vi "Example Indicator.vi"() -> ()   [LabVIEW 2010]
uses:
  C:/tf/play/labview/Tinkerforge.dll
  Tinkerforge.dll
panel:
  in  "uid":string="amb"
  in  "port":i32=4223
  in  "host":string="localhost"
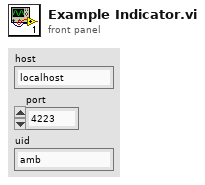
[diagram p1: front panel]
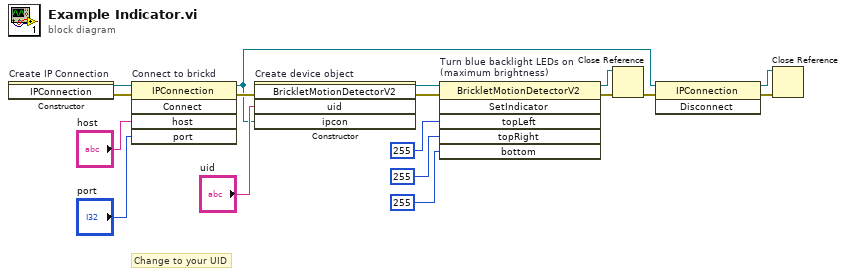
[diagram p0: block diagram]
diagram:
  # "Change to your UID"
  n1 = constructor on="Create IP Connection" class="IPConnection"() -> (reference out=w17:refnum<k24>, error out=w4:errorcluster)  [unwired: 3 in, 1 out]
  n2 = invoke on="Connect to brickd" class="IPConnection" method="Connect"(reference=w17, error in=w4, "host"="host", "port"="port") -> (reference out=w6:refnum<k24>, error out=w13:errorcluster)  [unwired: 1 in, 3 out]
  n3 = constructor on="Create device object" class="BrickletMotionDetectorV2"(error in=w13, "uid"="uid", "ipcon"=w6) -> (reference out=w11:refnum<k24>, error out=w12:errorcluster)  [unwired: 2 in, 3 out]
  n4 = invoke on="Turn blue backlight LEDs on\n(maximum brightness)" class="BrickletMotionDetectorV2" method="SetIndicator"(reference=w11, error in=w12, "topLeft"=u8 255, "topRight"=u8 255, "bottom"=u8 255) -> (reference out=w9:refnum<k24>, error out=w10:errorcluster)  [unwired: 1 in, 4 out]
  n5 = Close Reference(reference=w9, error in (no error)=w10) -> (error out=w8:errorcluster)
  n6 = invoke class="IPConnection" method="Disconnect"(reference=w6, error in=w8) -> (reference out=w5:refnum<k24>, error out=w7:errorcluster)  [unwired: 1 in, 1 out]
  n7 = Close Reference(reference=w5, error in (no error)=w7) -> ()  [unwired: 1 out]
